vi "Read Pin Map Context.vi"(8 "error in (no error)":errorcluster, 11 "MeasurementContext in":refnum<class "MeasurementContext.lvclass">) -> (0 "error out":errorcluster, 2 "pin map context":T1, 3 "MeasurementContext out":refnum<class "MeasurementContext.lvclass">)   [LabVIEW 2020, in "LineRegulation.lvlib" / "MeasurementContext.lvclass"]
uses:
  MeasurementContext.lvclass
  RPC Messages/ni_measurementlink_PinMapContext.ctl
  MeasurementContext.lvclass/MeasurementContext.ctl
  LineRegulation.lvlib
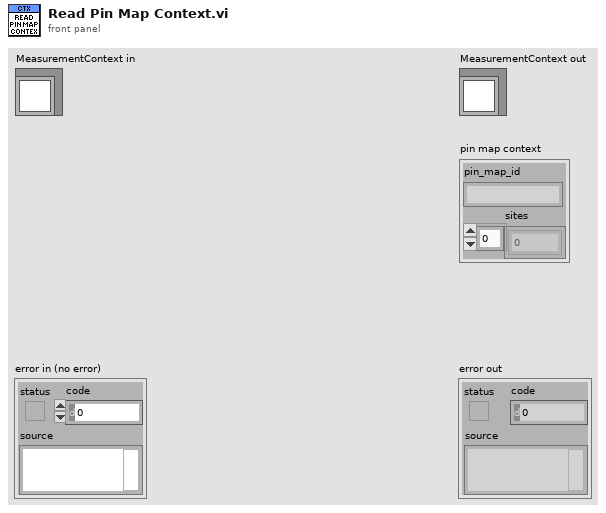
[diagram p1: front panel]
types:
  T1 = typedef "LineRegulation.lvlib/ni_measurementlink_PinMapContext.ctl" = cluster{"pin_map_id":string, "sites":i32[]}
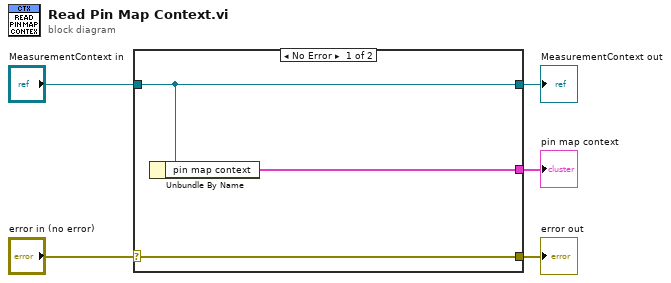
[diagram p0: block diagram]
diagram:
  n1 = case shown="No Error" "error in (no error)" {
    selector: "error in (no error)" -> [w8 w9]
    tunnel: [w8 w9] -> w4
    tunnel: [w7 w10] -> w2
    tunnel: "MeasurementContext in" -> [w7 w10]
    tunnel: [w6 _] -> w1
    frame No Error {
      n2 = Unbundle By Name(w7) -> ("pin map context"=w6:T1)
    }
    frame Error {
    }
  }
  "error out" <- w4
  "MeasurementContext out" <- w2
  "pin map context" <- w1
